vi "2psk.vi"() -> ()   [LabVIEW 2014]
uses:
  <vilib>/Analysis/NI_AALPro.lvlib
panel:
  out "modul":dynamicdata(graph)
  out "dig.data":dbl[](graph)
  out "demod":dynamicdata(graph)
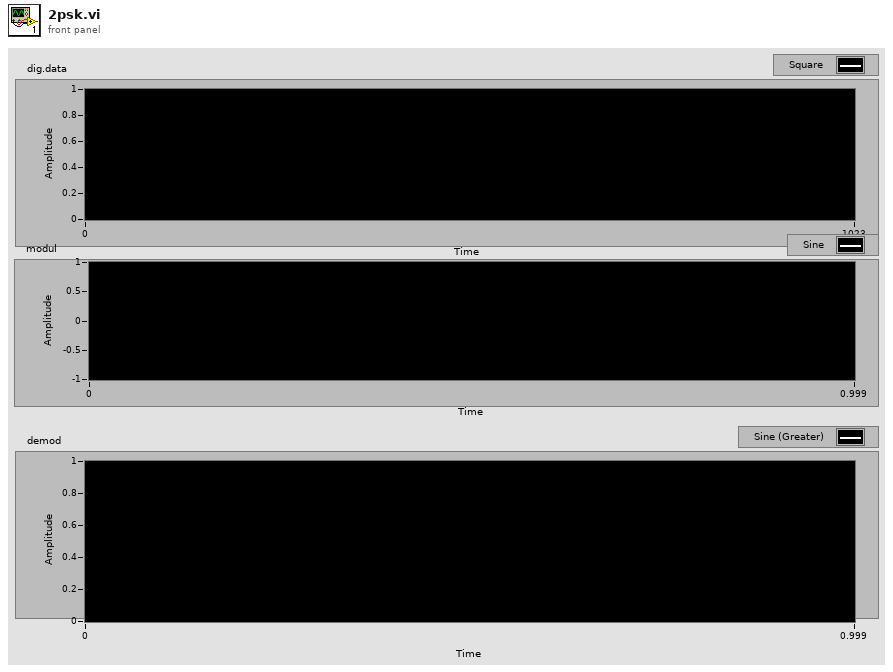
[diagram p1: front panel]
types:
  T1 = enum16{"sine", "cosine", "triangle", "square", "sawtooth", "increasing ramp", "decreasing ramp"}
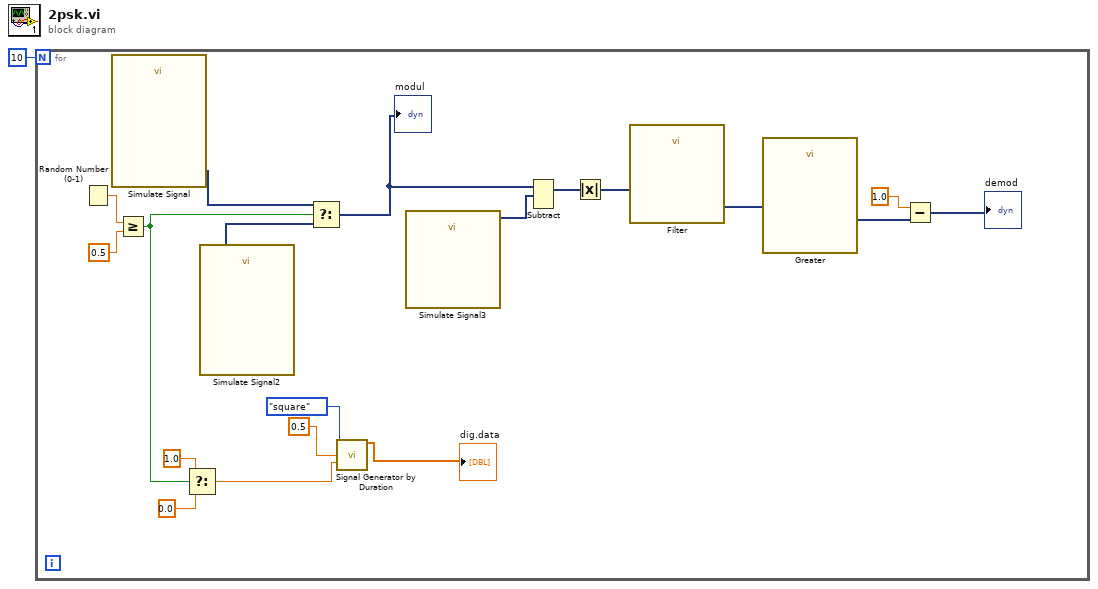
[diagram p0: block diagram]
diagram:
  n1 = for {
    N: 10 -> [_]
    n2 = Random Number (0-1)() -> (number: 0 to 1=w20:dbl)
    n3 = call "Simulate Signal"() -> ("Sine"=w16:dynamicdata)  [unwired: 14 in, 1 out]
    n4 = Greater Or Equal?(x=w20, y=0.5) -> (x >= y?=w14:bool)
    n5 = Select(t=1.0, s=w14, f=0.0) -> (s? t:f=w11:dbl)
    n6 = call "Simulate Signal2"() -> ("Sine"=w15:dynamicdata)  [unwired: 14 in, 1 out]
    n7 = Select(t=w16, s=w14, f=w15) -> (s? t:f=w9:dynamicdata)
    "modul" <- w9
    n8 = call <vilib>:"Signal Generator by Duration.vi"("signal type"=T1."square", "frequency"=0.5, "amplitude"=w11) -> ("signal"=→"dig.data":dbl[])  [unwired: 9 in, 3 out]
    n9 = call "Simulate Signal3"() -> ("Sine"=w8:dynamicdata)  [unwired: 14 in, 1 out]
    n10 = Subtract(1:w8, 2:w9) -> (0:w7:dynamicdata)  [unwired: 1 in, 1 out]
    n11 = Absolute Value(x=w7) -> (abs(x)=w6:dynamicdata)
    n12 = call "Filter"("Signal"=w6) -> ("Filtered Signal"=w5:dynamicdata)  [unwired: 9 in, 1 out]
    n13 = call "Greater"("Operand 1"=w5) -> ("Result"=w3:dynamicdata)  [unwired: 9 in, 1 out]
    n14 = Subtract(x=1.0, y=w3) -> (x-y=→"demod":dynamicdata)
  }
